vi "Set All Possible Connections.vi"(8 "error in (no error)":errorcluster, 10 "Possible Connections":T1[](array[typedef]), 11 "Hardware Ref in":T2 format="%.0x") -> (0 "error out":errorcluster, 3 "Hardware Ref out":T2 format="%.0x")   [LabVIEW 2020, in "Routing and Faulting Hardware API.lvlib"]
uses:
  Routing and Faulting Hardware API.lvlib
  <vilib>/NI VeriStand/Custom Device API/Custom Device Item Ref.ctl
  Types/Possible Connections for Endpoint.ctl
  NationalInstruments.VeriStand.SystemDefinitionAPI
  Routing and Faulting Hardware API Constants.vi
  <vilib>/NI VeriStand/Custom Device API/Custom Device API.lvlib
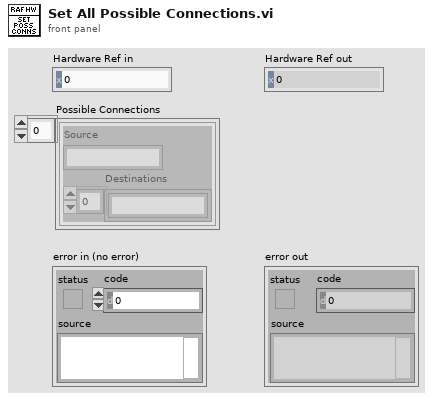
[diagram p1: front panel]
types:
  T1 = typedef "Routing and Faulting Hardware API.lvlib/Possible Connections for Endpoint.ctl" = cluster{"Source":string, "Destinations":string[]}
  T2 = typedef "Custom Device API.lvlib/Custom Device Item Ref.ctl" = u64
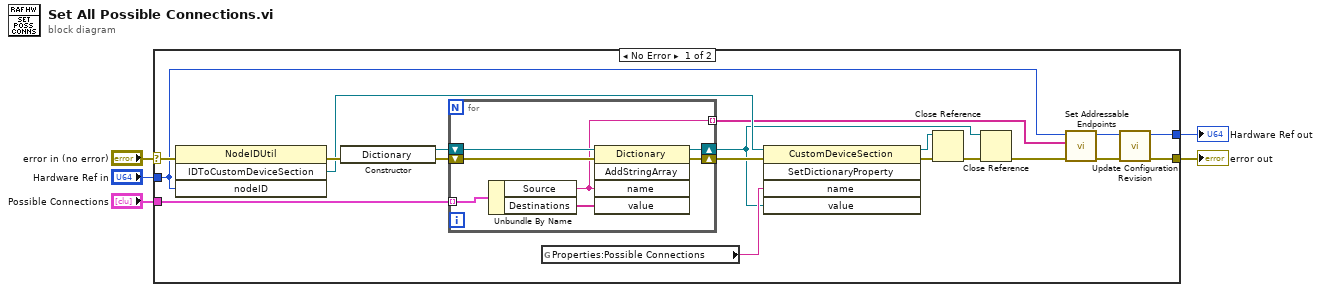
[diagram p0: block diagram]
diagram:
  n1 = case shown="No Error" "error in (no error)" {
    selector: "error in (no error)" -> [w18 w33]
    tunnel: [w8 w33] -> w5
    tunnel: "Hardware Ref in" -> [w12 w32]
    tunnel: [w7 w32] -> w2
    tunnel: "Possible Connections" -> [w17 _]
    frame No Error {
      n2 = invoke class="NodeIDUtil" method="IDToCustomDeviceSection"(error in=w18, "nodeID"=w12) -> (error out=w24:errorcluster, "IDToCustomDeviceSection"=w20:refnum<k24>)  [unwired: 2 in, 2 out]
      n3 = constructor class="Dictionary"(error in=w24) -> (reference out=w23:refnum<k24>, error out=w22:errorcluster)  [unwired: 2 in, 1 out]
      n4 = for {
        shift-right: [w29] -> w21
        shift-left: w22 -> [w30]
        shift-right: [w28] -> w13
        shift-left: w23 -> [w31]
        tunnel: w17 -> [w26] mode=indexing
        tunnel: [w25] -> w10 mode=indexing
        n5 = Unbundle By Name(w26) -> ("Source"=w25:string, "Destinations"=w27:string[])
        n6 = invoke class="Dictionary" method="AddStringArray"(reference=w31, error in=w30, "name"=w25, "value"=w27) -> (reference out=w28:refnum<k24>, error out=w29:errorcluster)  [unwired: 1 in, 3 out]
      }
      n7 = global read "Routing and Faulting Hardware API Constants.vi" "Properties:Possible Connections"() -> (w19:string)
      n8 = invoke class="CustomDeviceSection" method="SetDictionaryProperty"(reference=w20, error in=w21, "name"=w19, "value"=w13) -> (reference out=w15:refnum<k24>, error out=w16:errorcluster)  [unwired: 1 in, 3 out]
      n9 = Close Reference(reference=w15, error in (no error)=w16) -> (error out=w14:errorcluster)
      n10 = Close Reference(reference=w13, error in (no error)=w14) -> (error out=w11:errorcluster)
      n11 = call "Set Addressable Endpoints.vi"("error in (no error)"=w11, "Addressable Endpoints"=w10, "Hardware Ref in"=w12) -> ("error out"=w9:errorcluster, "Hardware Ref out"=w6:T2)  [unwired: 7 in]
      n12 = call "Update Configuration Revision.vi"("error in (no error)"=w9, "Hardware Ref in"=w6) -> ("error out"=w8:errorcluster, "Hardware Ref out"=w7:T2)  [unwired: 8 in]
    }
    frame Error {
    }
  }
  "Hardware Ref out" <- w2
  "error out" <- w5
